vi "action.vi"(0 "HGF_FGV_Append":refnum<class "HGF_FGV_Replace.lvclass">, 2 "Objects":refnum<class>[](array[class]), 5 "error in (no error)":errorcluster) -> (14 "dup HGF_FGV_Append":refnum<class "HGF_FGV_Replace.lvclass">, 16 "dup Objects":refnum<class>[](array[class]), 19 "error out":errorcluster)   [LabVIEW 2012, in "HGF_FGV.lvlib" / "HGF_FGV_Replace.lvclass"]
doc: "Replace object array at index."
uses:
  HGF_FGV_Replace.lvclass
  HGF_FGV_Replace.lvclass/HGF_FGV_Replace.ctl
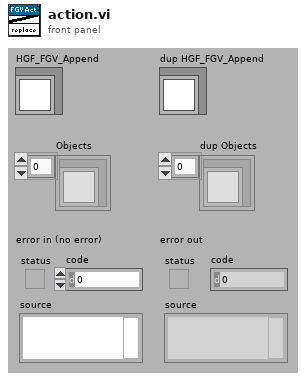
[diagram p1: front panel]
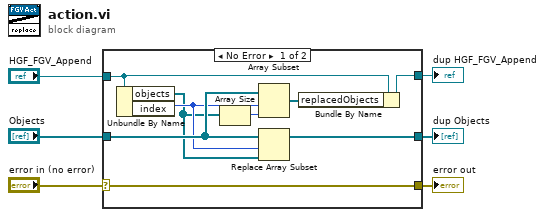
[diagram p0: block diagram]
diagram:
  n1 = case shown="No Error" "error in (no error)" {
    selector: "error in (no error)" -> [w15 w18]
    tunnel: [w15 w18] -> w5
    tunnel: [w8 w17] -> w3
    tunnel: "HGF_FGV_Append" -> [w9 w17]
    tunnel: [w14 w16] -> w2
    tunnel: "Objects" -> [w13 w16]
    frame No Error {
      n2 = Unbundle By Name(w9) -> ("objects"=w11:refnum<class>[], "index"=w12:i32)
      n3 = Array Size(array=w11) -> (size(s)=w10:i32)
      n4 = Array Subset(array=w13, index=w12, length=w10) -> (w7:refnum<class>[])
      n5 = Replace Array Subset(array=w13, new element=w11, index=w12) -> (w14:refnum<class>[])
      n6 = Bundle By Name(cluster=w9, "replacedObjects"=w7) -> (w8:refnum<class "HGF_FGV_Replace.lvclass">)
    }
    frame Error {
    }
  }
  "error out" <- w5
  "dup HGF_FGV_Append" <- w3
  "dup Objects" <- w2
